vi "Queue Nested Status.vi"(11 "Actor in":refnum<class "Actor.lvclass">) -> (0 "Queue Nested Count":i32, 1 "Queue Nested Aliases":string[](array[string]), 2 "Any Exist?":bool)   [LabVIEW 2021, in "jettl.lvlib" / "Actor.lvclass"]
uses:
  Actor.lvclass
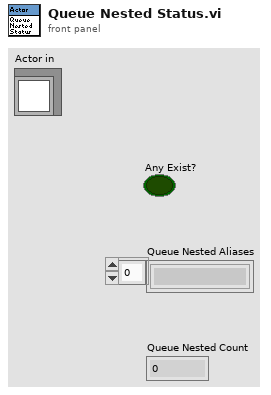
[diagram p1: front panel]
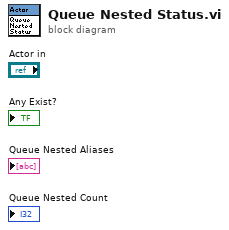
[diagram p0: block diagram]
diagram:
